vi "Vent To Atmosphere.vi"(8 "error in (no error)":errorcluster) -> (0 "error out":errorcluster)   [LabVIEW 2018]
uses:
  Valve Globals.vi
panel:
  in  "4 - close 6":bool[](array[boolean])=[TRUE, TRUE, FALSE, FALSE, TRUE, FALSE, TRUE, FALSE, FALSE, FALSE, FALSE, FALSE]
  in  "3 - open\n1 and 2":bool[](array[boolean])=[TRUE, TRUE, FALSE, FALSE, TRUE, TRUE, TRUE, FALSE, FALSE, FALSE, FALSE, FALSE]
  in  "2 - open \n5 and 7":bool[](array[boolean])=[FALSE, FALSE, FALSE, FALSE, TRUE, TRUE, TRUE, FALSE, FALSE, FALSE, FALSE, FALSE]
  in  "1 - only \n6 open":bool[](array[boolean])=[FALSE, FALSE, FALSE, FALSE, FALSE, TRUE, FALSE, FALSE, FALSE, FALSE, FALSE, FALSE]
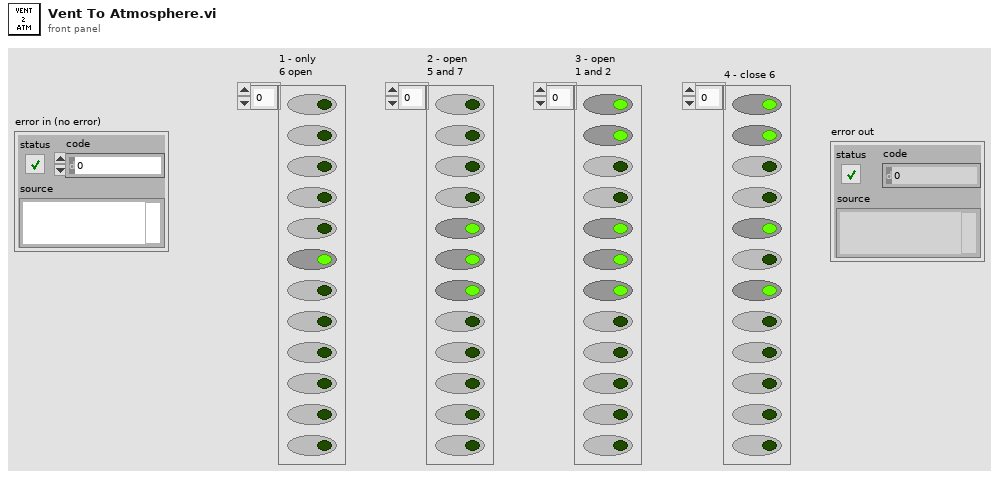
[diagram p1: front panel]
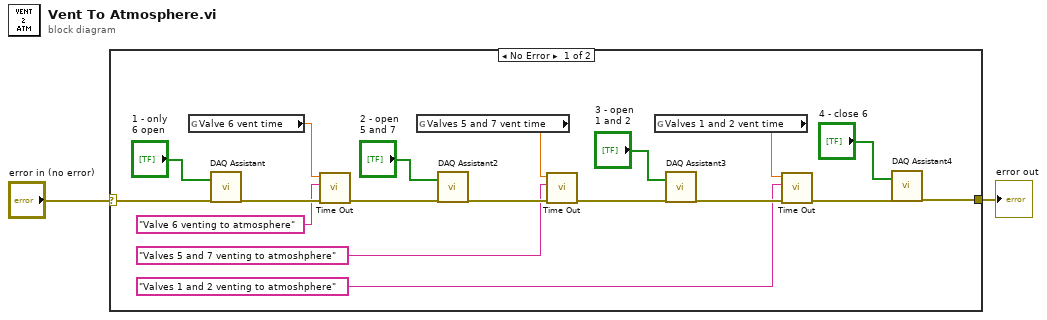
[diagram p0: block diagram]
diagram:
  n1 = case shown="No Error" "error in (no error)" {
    selector: "error in (no error)" -> [w6 w21]
    tunnel: [w7 w21] -> w2
    frame No Error {
      n2 = global read "Valve Globals.vi" "Valve 6 vent time"() -> (w20:dbl)
      n3 = call "DAQ Assistant"("data"="1 - only \n6 open", "error in"=w6) -> ("error out"=w18:errorcluster)  [unwired: 16 in, 1 out]
      n4 = call "Time Out.vi"("error in (no error)"=w18, 10:"Valve 6 venting to atmosphere", "Numeric"=w20) -> ("error out"=w16:errorcluster)  [unwired: 8 in]
      n5 = global read "Valve Globals.vi" "Valves 5 and 7 vent time"() -> (w14:dbl)
      n6 = call "DAQ Assistant2"("data"="2 - open \n5 and 7", "error in"=w16) -> ("error out"=w15:errorcluster)  [unwired: 16 in, 1 out]
      n7 = call "Time Out.vi"("error in (no error)"=w15, 10:"Valves 5 and 7 venting to atmoshphere", "Numeric"=w14) -> ("error out"=w11:errorcluster)  [unwired: 8 in]
      n8 = global read "Valve Globals.vi" "Valves 1 and 2 vent time"() -> (w12:dbl)
      n9 = call "DAQ Assistant3"("data"="3 - open\n1 and 2", "error in"=w11) -> ("error out"=w10:errorcluster)  [unwired: 16 in, 1 out]
      n10 = call "Time Out.vi"("error in (no error)"=w10, 10:"Valves 1 and 2 venting to atmoshphere", "Numeric"=w12) -> ("error out"=w8:errorcluster)  [unwired: 8 in]
      n11 = call "DAQ Assistant4"("data"="4 - close 6", "error in"=w8) -> ("error out"=w7:errorcluster)  [unwired: 16 in, 1 out]
    }
    frame Error {
    }
  }
  "error out" <- w2
